vi "FMA1600A Bus Data Filter.vi"(0 "Station A Input":string, 1 "Station B Input":string, 2 "Station C Input":string, 3 "Station D Input":string, 4 "Station E Input":string, 5 "Error In":errorcluster, 6 "Unit ID":string, 7 "Station F Input":string, 8 "Data Stream":string, 9 "FMA1600A Gas Data":T1) -> (11 "Check Shutdown":bool, 13 "Station F Output":string, 14 "Station A Output":string, 15 "Station B Output":string, 16 "Station C Output":string, 17 "Station D Output":string, 18 "Station E Output":string, 19 "Error Out":errorcluster)   [LabVIEW 2018]
uses:
  Type Definitions/FMA1600A Data.ctl
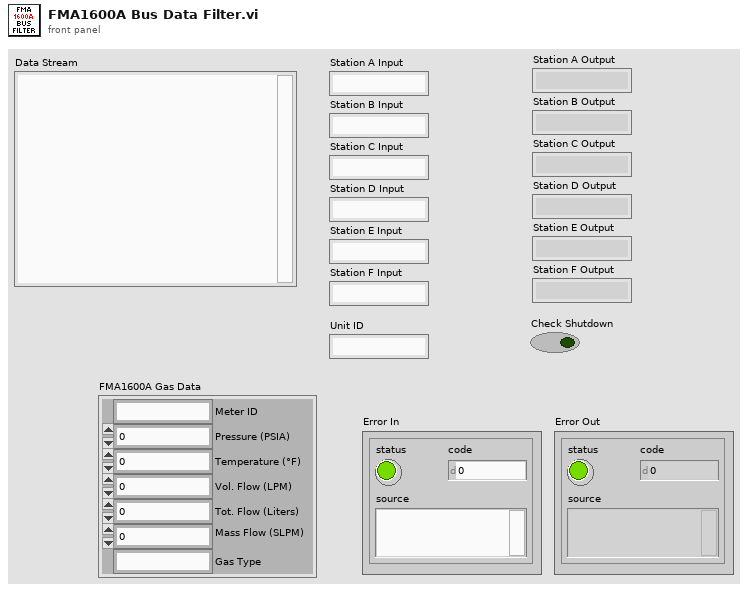
[diagram p1: front panel]
types:
  T1 = typedef "FMA1600A Data.ctl" = cluster{"Pressure (PSIA)":dbl, "Temperature (°F)":dbl, "Vol. Flow (LPM)":dbl, "Mass Flow (SLPM)":dbl, "Gas Type":string, "Tot. Flow (Liters)":dbl, "Meter ID":string}
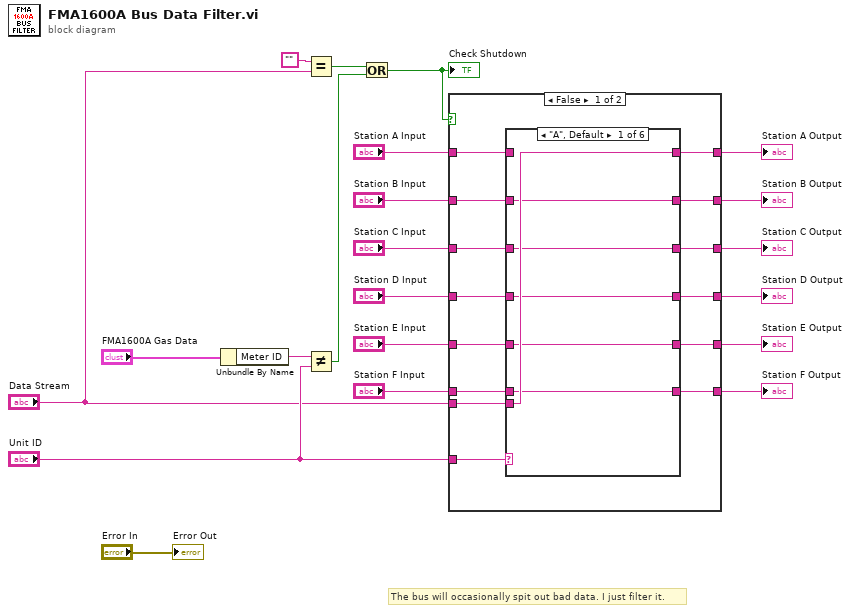
[diagram p0: block diagram]
diagram:
  # "The bus will occasionally spit out bad data. I just filter it."
  n1 = Unbundle By Name("FMA1600A Gas Data") -> ("Meter ID"=w17:string)
  n2 = Equal?(x="", y="Data Stream") -> (x = y?=w18:bool)
  n3 = Not Equal?(x=w17, y="Unit ID") -> (x != y?=w19:bool)
  n4 = Or(x=w18, y=w19) -> (x .or. y?=w20:bool)
  "Check Shutdown" <- w20
  n5 = case shown="False" w20 {
    tunnel: "Unit ID" -> [w35 _]
    tunnel: "Data Stream" -> [w34 _]
    tunnel: [w33 w77] -> w2
    tunnel: [w32 w76] -> w3
    tunnel: [w31 w75] -> w4
    tunnel: [w30 w74] -> w5
    tunnel: [w29 w73] -> w6
    tunnel: [w28 w72] -> w7
    tunnel: "Station B Input" -> [w27 w77]
    tunnel: "Station C Input" -> [w26 w76]
    tunnel: "Station F Input" -> [w25 w75]
    tunnel: "Station E Input" -> [w24 w74]
    tunnel: "Station D Input" -> [w23 w73]
    tunnel: "Station A Input" -> [w22 w72]
    frame False {
      n6 = case shown="\"A\", Default" w35 {
        tunnel: [w40 w47 w51 w57 w63 w71] -> w33
        tunnel: w34 -> [w41 w47 w53 w59 w62 w67]
        tunnel: [w39 w45 w53 w56 w65 w70] -> w32
        tunnel: [w36 w42 w48 w54 w60 w67] -> w31
        tunnel: [w37 w43 w49 w55 w62 w69] -> w30
        tunnel: [w38 w44 w50 w59 w61 w68] -> w29
        tunnel: [w41 w46 w52 w58 w64 w66] -> w28
        tunnel: w27 -> [w40 _ w51 w57 w63 w71]
        tunnel: w26 -> [w39 w45 _ w56 w65 w70]
        tunnel: w25 -> [w36 w42 w48 w54 w60 _]
        tunnel: w24 -> [w37 w43 w49 w55 _ w69]
        tunnel: w23 -> [w38 w44 w50 _ w61 w68]
        tunnel: w22 -> [_ w46 w52 w58 w64 w66]
        frame "A", Default {
        }
        frame "B" {
        }
        frame "C" {
        }
        frame "D" {
        }
        frame "E" {
        }
        frame "F" {
        }
      }
    }
    frame True {
    }
  }
  "Station A Output" <- w7
  "Station D Output" <- w6
  "Station E Output" <- w5
  "Station F Output" <- w4
  "Station C Output" <- w3
  "Station B Output" <- w2
  "Error Out" <- "Error In"
